vi "UsrProfiles-Export profile dialogue.vi"(8 "error in (no error)":errorcluster, 11 "Profile's file path":path) -> (0 "error out":errorcluster, 2 "cancelled":bool, 3 "selected path":path)   [LabVIEW 2020]
uses:
  <userlib>/_MGI/File/MGI Windows Folder Enum.ctl
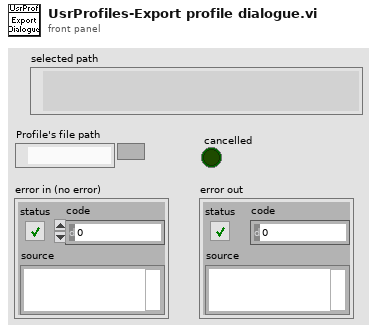
[diagram p1: front panel]
types:
  T1 = typedef "MGI Windows Folder Enum.ctl" = enum32{"Desktop", "Err<Internet>", "Programs", "Err<Controls>", "Err<Printers>", "Personal (MyDocuments)", "Favorites", "Startup", "Recent", "SendTo", "Err<RecycleBin>", "StartMenu", "Err<MyDocuments>", "MyMusic", "MyVideo", "Err<0x000F>", "DesktopDirectory", "Err<Drives>", "Err<Network>", "NetHood", "Fonts", "Templates", "CommonStartMenu", "CommonPrograms", "CommonStartup", "CommonDesktopDirectory", "AppData", "PrintHood", "LocalAppData", "Err<AltStartup>", "Err<CommonAltStartup>", "CommonFavorites", "InternetCache", "Cookies", "History", "CommonAppData", "Windows", "System", "ProgramFiles", "MyPictures", "Profile", "System32", "Err<0x002A>", "ProgramFilesCommon", "Err<0x002C>", "CommonTemplates", "CommonDocuments", "CommonAdminTools", "AdminTools"}
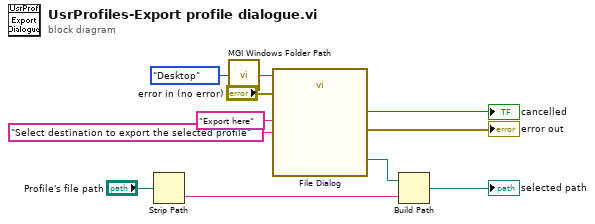
[diagram p0: block diagram]
diagram:
  n1 = Strip Path(path="Profile's file path") -> (name=w3:string)  [unwired: 1 out]
  n2 = call <userlib>:"MGI Windows Folder Path.vi"("Windows Folder"=MGI_Windows_Folder_Enum."Desktop") -> ("Path"=w6:path)
  n3 = call "File Dialog"("start path"=w6, "prompt"="Select destination to export the selected profile", "button label"="Export here", "error in"="error in (no error)") -> ("selected path"=w2:path, "cancelled"=→"cancelled":bool, "error out"=→"error out":errorcluster)  [unwired: 8 in, 1 out]
  n4 = Build Path(base path=w2, name or relative path=w3) -> (appended path=→"selected path":path)
